vi "SSS_V3.0.vi"() -> ()   [LabVIEW 2017]
uses:
  <vilib>/DAQmx/write.llb/DAQmx Write (Analog 2D DBL NChan NSamp).vi
  <vilib>/DAQmx/read.llb/DAQmx Read (Analog 1D Wfm NChan NSamp).vi
  <vilib>/DAQmx/create/channels.llb/DAQmx Create Channel (AO-Voltage-Basic).vi
  <vilib>/DAQmx/create/channels.llb/DAQmx Create Channel (AI-Voltage-Basic).vi
  <vilib>/DAQmx/configure/timing.llb/DAQmx Timing (Sample Clock).vi
  <vilib>/DAQmx/miscellaneous.llb/DAQmx Fill In Error Info.vi
panel:
  out "배열":i32[](array[numeric])
  in  "physical channels":tag="Dev3/ao0:1" caption="송신 채널 설정"
  in  "Samplig Rate(RX)":dbl=1500000.0
  in  "RX time(sec)":dbl=0.1
  out "RX.CH2 2":waveform(dbl)(graph)
  out "RX.CH2":waveform(dbl)(graph)
  in  "Start Frequency(Hz)":dbl=430000.0 format="%#_6p"
  in  "Pulse length(sec)":dbl=4e-06 format="%#_6p"
  in  "sampling rate(TX)":dbl=3760000.0 caption="Sampling Rate(TX)" format="%#.2g"
  in  "STEP":i32=100
  in  "초기 위상":dbl format="%#_13g"
  in  "Bandwidth":dbl=40000.0 format="%#_6p"
  out "Hz/1STEP":dbl
  out "TX.CH1":waveform(dbl)(graph)
  out "TX Spectrum":cluster{"f0":dbl, "df":dbl, "magnitude":dbl[]}(graph)
  out "TX.CH 2":waveform(dbl)(graph)
  in  "수신 디바이스 이름":tag="Dev3"
  in  "수신 채널 설정":tag="Dev3/ai0:1"
  in  "Number of Sample":i32=150000 format="%#.0g"
  in  "송신 디바이스 이름":tag="Dev3"
  out "불리언 2":bool
  in  "Signal_Processing 2":bool
  out "CMD_PWD_DATA":i32=4
  in  "Signal_Processing":bool
  out "CMD_PWD":i32=7
  out "CMD_TVG":i32=6
  out "CMD_TVG_DATA":i32=4
  out "CMD_GAIN":i32=5
  out "CMD_GAIN_DATA":i32=255
  out "CMD_RANGE":i32=4
  out "CMD_RANGE_DATA":i32=100
  out "CMD_STOP":i32=3
  out "CMD_STOP_DATA":i32
  out "CMD_START":i32=2
  out "CMD_START_DATA":i32=1
  in  "port":u16=2500
  in  "address":string="30.0.1.18"
  in  "TCP/IP":bool
  in  "Server Closed":string="The server VI closed the connection."
  # "송신 신호 변조 설정"
  # "DAQ Max 설정"
  # "TCP/IP 소켓 통신 설정"
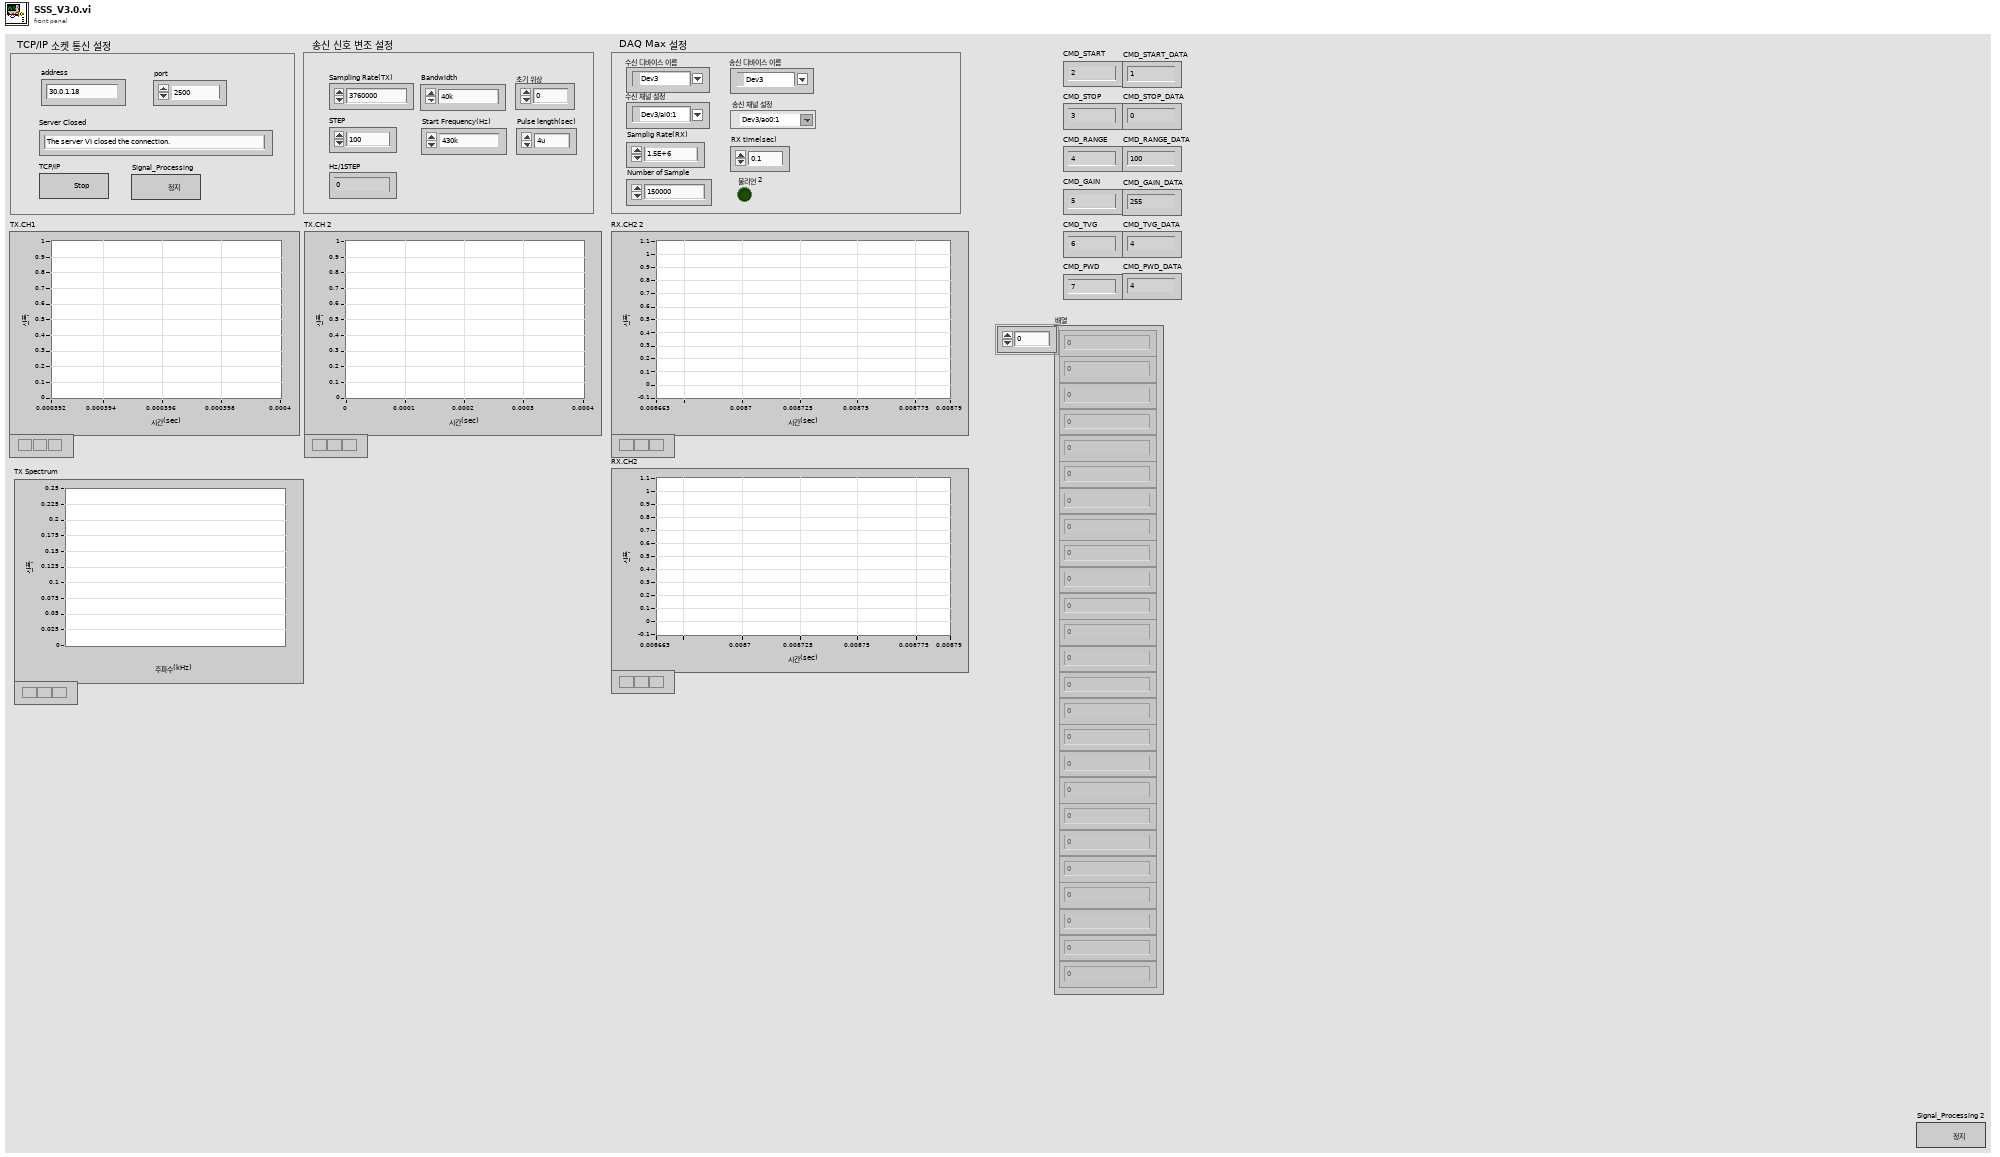
[diagram p1: front panel]
types:
  T1 = enum16{"Standard", "Buffered", "CRLF", "Immediate"}
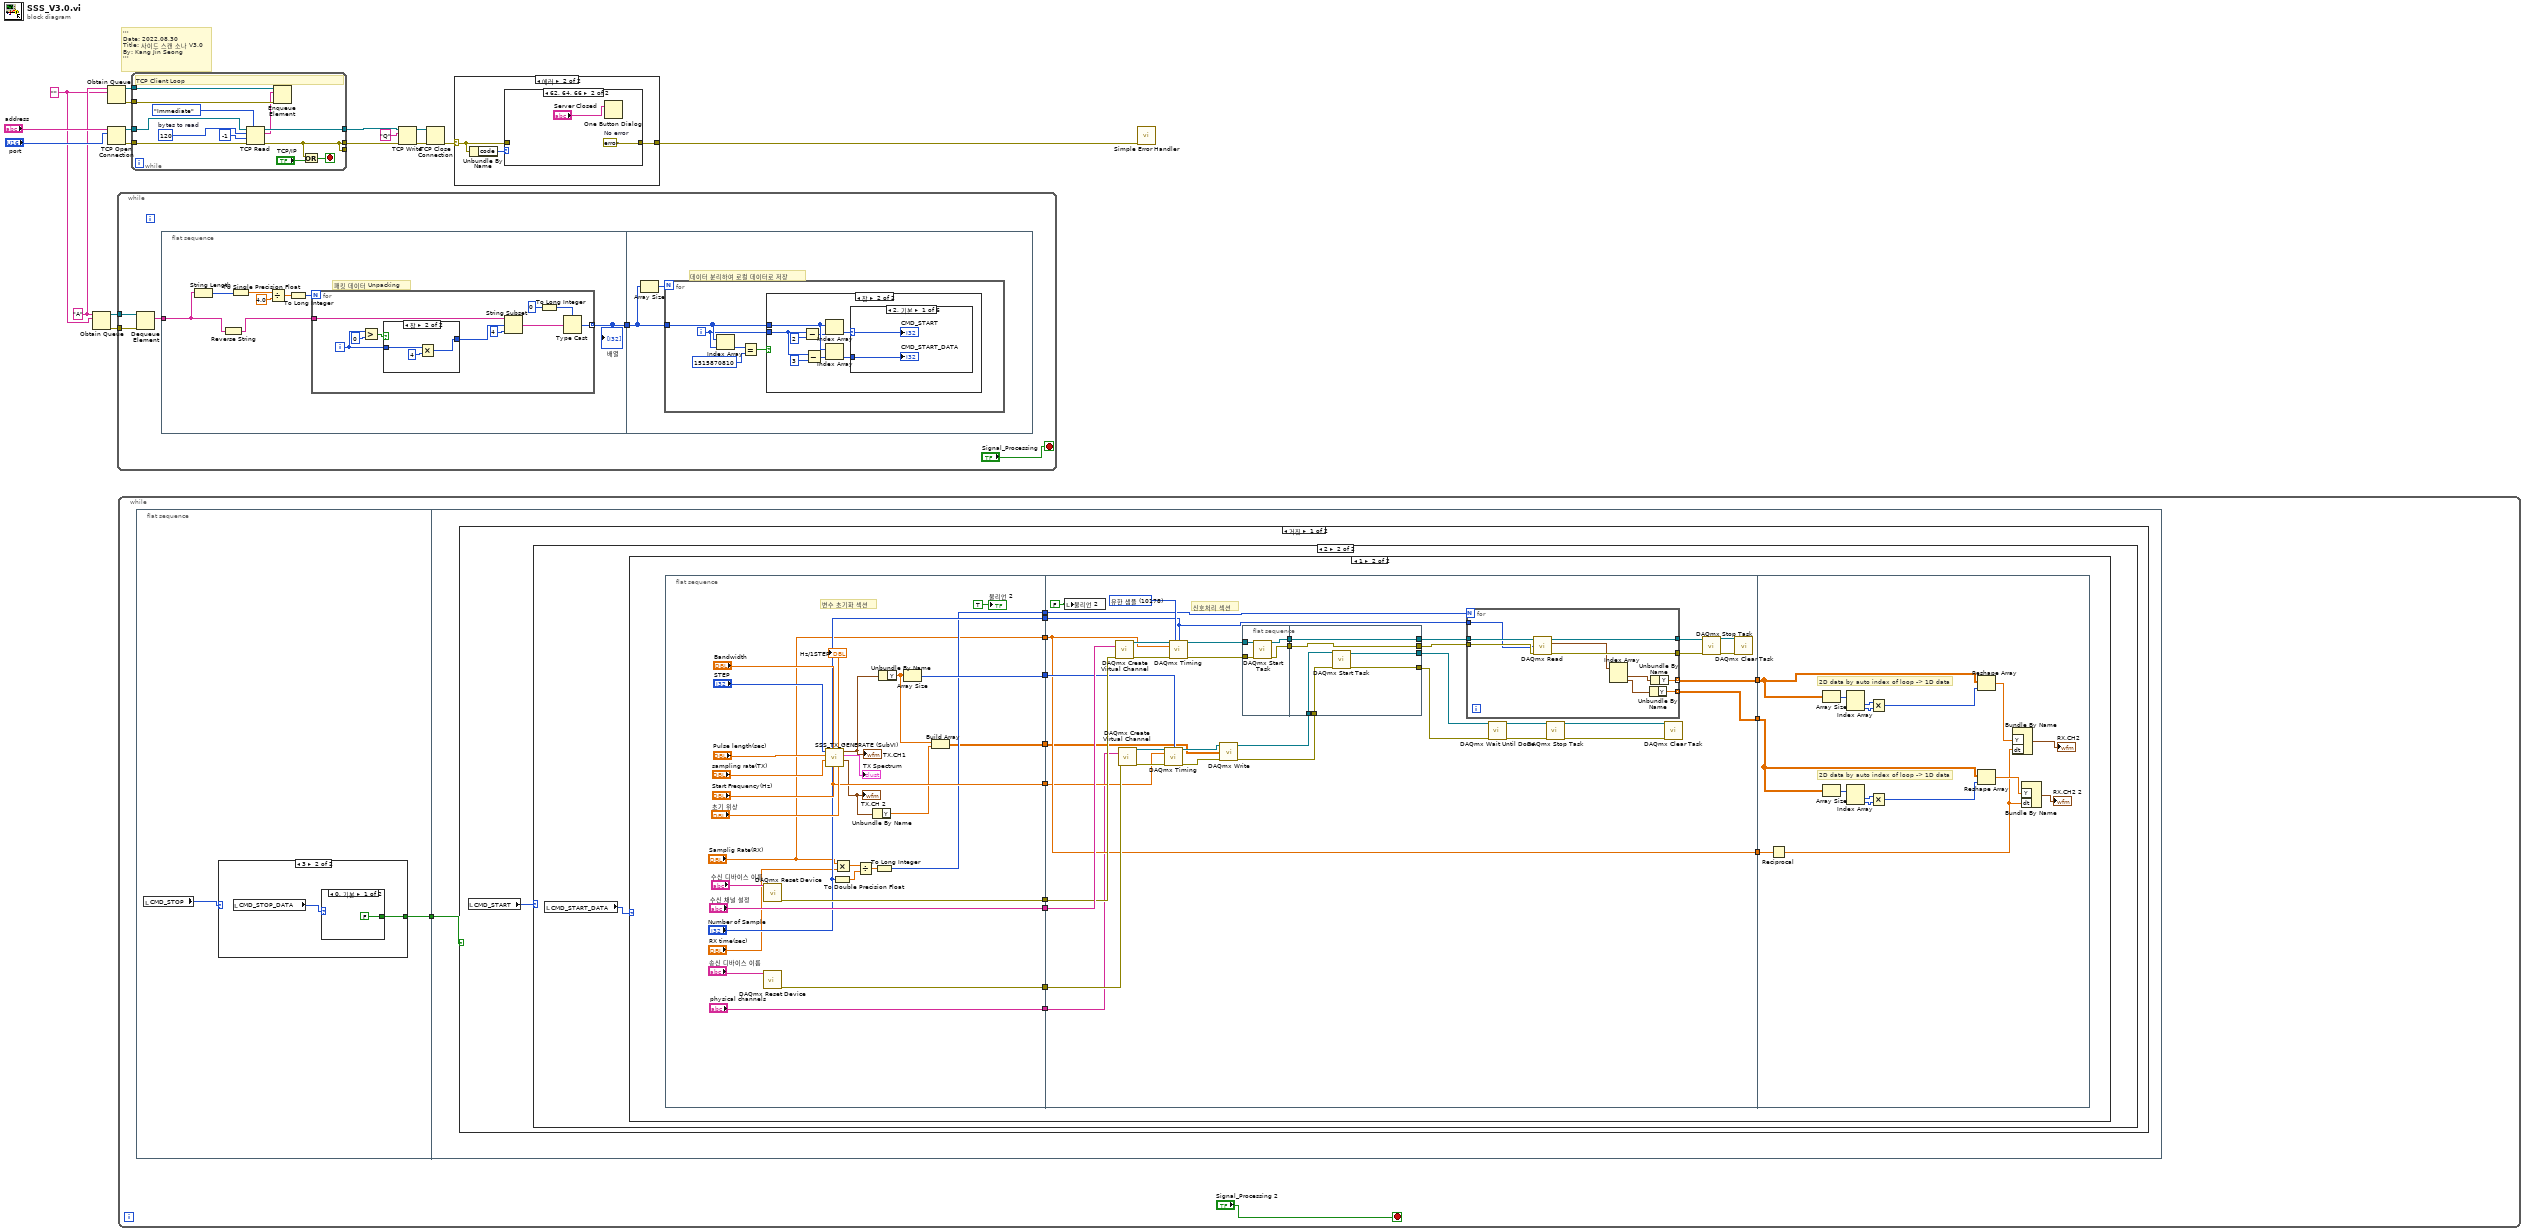
[diagram p0: block diagram]
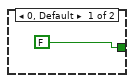
[diagram p2: hidden frame]
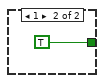
[diagram p3: hidden frame]
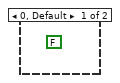
[diagram p4: hidden frame]
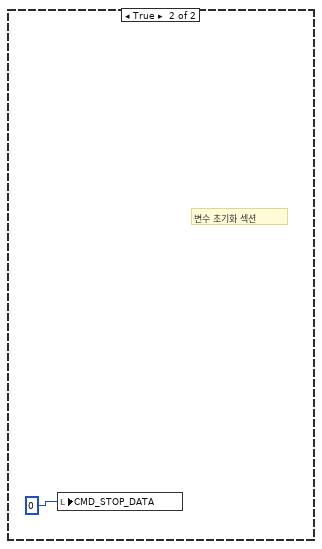
[diagram p6: hidden frame]
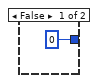
[diagram p7: hidden frame]
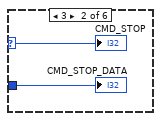
[diagram p9: hidden frame]
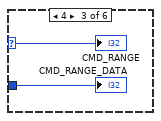
[diagram p10: hidden frame]
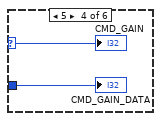
[diagram p11: hidden frame]
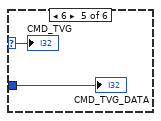
[diagram p12: hidden frame]
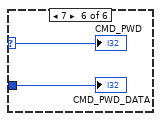
[diagram p13: hidden frame]
diagram:
  w1 = ""
  w4 = "A" ("이름(이름없음)")
  # "'''\nDate: 2022.08.30\nTitle: 사이드 스캔 소나 V3.0\nBy: Kang Jin Seong\n'''"
  n1 = Obtain Queue(name (unnamed)=w4, element data type=w1) -> (queue out=w3:refnum<queue>, error out=w2:errorcluster)  [unwired: 3 in, 1 out]
  n2 = Obtain Queue(name (unnamed)=w4, element data type=w1) -> (queue out=w6:refnum<queue>, error out=w5:errorcluster)  [unwired: 3 in, 1 out]
  n3 = TCP Open Connection(address="address", remote port or service name="port") -> (connection ID=w7:refnum<k5>, error out=w8:errorcluster)  [unwired: 3 in]
  n4 = while {
    tunnel: w3 -> [w21]
    tunnel: w2 -> [w20]
    stop <- "Signal_Processing" stop-if-true
    n5 = Dequeue Element(queue=w21, error in (no error)=w20) -> (element=w19:string)  [unwired: 1 in, 3 out]
    n6 = flat-sequence {
      tunnel: w19 -> [w24]
      tunnel: [w25] -> w22
      tunnel: w22 -> [w45]
      frame #0 {
        # "패킷 데이터 Unpacking"
        n7 = String Length(string=w24) -> (length=w30:i32)
        n8 = Reverse String(1:w24) -> (0:w23:string)
        n9 = To Single Precision Float(number=w30) -> (single precision float=w29:sgl)
        n10 = Divide(x=w29, y=sgl 4.0) -> (x/y=w27:sgl)
        n11 = To Long Integer(number=w27) -> (32bit integer=w26:i32)
        n12 = for {
          N: w26 -> [_]
          tunnel: w23 -> [w40]
          tunnel: [w37] -> w25 mode=indexing
          i -> [w32]
          n13 = Greater?(x=w32, y=0) -> (0:w34:bool)
          n14 = case shown="참" w34 {
            tunnel: [0 w42] -> w33
            tunnel: w32 -> [_ w44]
            frame False {
            }
            frame True {
              n15 = Multiply(x=w44, y=4) -> (x*y=w42:i32)
            }
          }
          n16 = String Subset(string=w40, offset (0)=w33, length (rest)=4 ("길이(나머지)")) -> (substring=w31:string)
          n17 = To Long Integer(number=0 ("숫자")) -> (32bit integer=w39:i32)
          n18 = Type Cast(type=w39, x=w31) -> (*(type *) &x=w37:i32)
        }
        "배열" <- w25
      }
      frame #1 {
        # "데이터 분리하여 로컬 데이터로 저장"
        n19 = Array Size(array=w45) -> (size(s)=w46:i32)
        n20 = for {
          N: w46 -> [_]
          tunnel: w45 -> [w48]
          i -> [w47]
          n21 = Index Array(array=w48, index=w47) -> (element=w51:i32)
          n22 = Equal?(x=w51, y=1515870810) -> (x = y?=w49:bool)
          n23 = case shown="참" w49 {
            tunnel: w48 -> [_ w58]
            tunnel: w47 -> [_ w54]
            frame False {
            }
            frame True {
              n24 = Subtract(x=w54, y=2) -> (x-y=w52:i32)
              n25 = Subtract(x=w54, y=3) -> (x-y=w55:i32)
              n26 = Index Array(array=w58, index=w52) -> (element=w59:i32)
              n27 = Index Array(array=w58, index=w55) -> (element=w57:i32)
              n28 = case shown="2, 기본" w59 {
                selector: w59 -> [w61 w63 w65 w67 w69 w71]
                tunnel: w57 -> [w60 w62 w64 w66 w68 w70]
                frame 2, Default {
                  "CMD_START" <- w61
                  "CMD_START_DATA" <- w60
                }
                frame 3 {
                  "CMD_STOP" <- w63
                  "CMD_STOP_DATA" <- w62
                }
                frame 4 {
                  "CMD_RANGE" <- w65
                  "CMD_RANGE_DATA" <- w64
                }
                frame 5 {
                  "CMD_GAIN" <- w67
                  "CMD_GAIN_DATA" <- w66
                }
                frame 6 {
                  "CMD_TVG" <- w69
                  "CMD_TVG_DATA" <- w68
                }
                frame 7 {
                  "CMD_PWD" <- w71
                  "CMD_PWD_DATA" <- w70
                }
              }
            }
          }
        }
      }
    }
  }
  n29 = while {
    stop <- "Signal_Processing 2" stop-if-true
    n30 = flat-sequence {
      tunnel: [w74] -> w72
      tunnel: w72 -> [w81]
      frame #0 {
        n31 = local read "CMD_STOP"() -> (w75:i32)
        n32 = case shown="3" w75 {
          tunnel: [FALSE w77] -> w74
          frame 0, Default {
          }
          frame 3 {
            n33 = local read "CMD_STOP_DATA"() -> (w78:i32)
            n34 = case shown="0, 기본" w78 {
              tunnel: [FALSE TRUE] -> w77
              frame 0, Default {
              }
              frame 1 {
              }
            }
          }
        }
      }
      frame #1 {
        n35 = case shown="거짓" w81 {
          frame False {
            n36 = local read "CMD_START"() -> (w82:i32)
            n37 = case shown="2" w82 {
              frame 0, Default {
                (unwired) FALSE
              }
              frame 2 {
                n38 = local read "CMD_START_DATA"() -> (w83:i32)
                n39 = case shown="1" w83 {
                  frame 0, Default {
                  }
                  frame 1 {
                    n40 = flat-sequence {
                      tunnel: ["Start Frequency(Hz)"] -> w96
                      tunnel: ["수신 채널 설정"] -> w95
                      tunnel: [w110] -> w94
                      tunnel: ["Samplig Rate(RX)"] -> w93
                      tunnel: ["Number of Sample"] -> w92
                      tunnel: [w108] -> w91
                      tunnel: [w106] -> w90
                      tunnel: [w105] -> w89
                      tunnel: [w100] -> w85
                      tunnel: ["physical channels"] -> w84
                      tunnel: [w138] -> w88
                      tunnel: w96 -> [w128]
                      tunnel: w95 -> [w136]
                      tunnel: w94 -> [w135]
                      tunnel: w93 -> [w130]
                      tunnel: w92 -> [w129]
                      tunnel: w91 -> [w133]
                      tunnel: w90 -> [w132]
                      tunnel: w89 -> [w131]
                      tunnel: [w130] -> w87
                      tunnel: [w127] -> w86
                      tunnel: w85 -> [w126]
                      tunnel: w84 -> [w125]
                      tunnel: w88 -> [w192]
                      tunnel: w87 -> [w191]
                      tunnel: w86 -> [w186]
                      frame #0 {
                        # "변수 초기화 섹션"
                        n41 = call <vilib>:"DAQmx Reset Device.vi"("device in"="송신 디바이스 이름") -> ("error out"=w105:errorcluster)  [unwired: 1 in, 13 out]
                        n42 = call <vilib>:"DAQmx Reset Device.vi"("device in"="수신 디바이스 이름") -> ("error out"=w110:errorcluster)  [unwired: 1 in, 13 out]
                        n43 = call "SSS_TX_GENERATE (SubVI).vi"("초기 위상"="초기 위상", "Start Frequency(Hz)"="Start Frequency(Hz)", "Bandwidth"="Bandwidth", "sampling rate"="sampling rate(TX)", "Pulse length(sec)"="Pulse length(sec)", "STEP"="STEP") -> ("TX.CH1 2"=w103:waveform(dbl), "TX Spectrum"=→"TX Spectrum":cluster{"f0":dbl, "df":dbl, "magnitude":dbl[]}, "TX.CH1"=w109:waveform(dbl), "Hz/1STEP"=→"Hz/1STEP":dbl)  [unwired: 2 in]
                        "TX.CH1" <- w109
                        "TX.CH 2" <- w103
                        n44 = To Double Precision Float(number="Number of Sample") -> (double precision float=w116:dbl)
                        n45 = Multiply(x="Samplig Rate(RX)", y="RX time(sec)") -> (x*y=w115:dbl)
                        n46 = Divide(x=w115, y=w116) -> (x/y=w117:dbl)
                        n47 = Unbundle By Name(w103) -> ("Y"=w101:dbl[])
                        n48 = To Long Integer(number=w117) -> (32bit integer=w106:i32)
                        n49 = Unbundle By Name(w109) -> ("Y"=w102:dbl[])
                        n50 = Array Size(array=w102) -> (size(s)=w108:i32)
                        n51 = Build Array(w102, w101) -> (w100:dbl[][])
                        "불리언 2" <- TRUE
                      }
                      frame #1 {
                        w134 = 10178 items=["유한 샘플"=10178, "연속 샘플"=10123, "하드웨어 타이밍에 의한 단일 포인트"=12522] ("sample mode")
                        # "신호처리 섹션"
                        n52 = local write "불리언 2"(FALSE) -> ()
                        n53 = call-poly <vilib>:"DAQmx Create Virtual Channel.vi"("physical channels"=w136, "error in"=w135) -> ("task out"=w159:refnum<k21>, "error out"=w160:errorcluster)  [unwired: 7 in, 5 out]
                        n54 = call-poly <vilib>:"DAQmx Create Virtual Channel.vi"("physical channels"=w125, "error in"=w131) -> ("task out"=w150:refnum<k21>, "error out"=w149:errorcluster)  [unwired: 7 in, 5 out]
                        n55 = call-poly <vilib>:"DAQmx Timing.vi"("task/channels in"=w150, "samples per channel"=w133, "rate"=w128, "error in"=w149) -> ("task out"=w147:refnum<k21>, "error out"=w148:errorcluster)  [unwired: 3 in, 7 out]
                        n56 = call-poly <vilib>:"DAQmx Timing.vi"("task/channels in"=w159, "sample mode"=w134, "samples per channel"=w129, "rate"=w130, "error in"=w160) -> ("task out"=w158:refnum<k21>, "error out"=w157:errorcluster)  [unwired: 2 in, 7 out]
                        n57 = call-poly <vilib>:"DAQmx Write.vi"("task/channels in"=w147, "data"=w126, "error in"=w148) -> ("task out"=w146:refnum<k21>, "error out"=w145:errorcluster)  [unwired: 10 in, 1 out]
                        n58 = flat-sequence {
                          tunnel: [w176] -> w162
                          tunnel: [w175] -> w161
                          tunnel: w158 -> [w174]
                          tunnel: w157 -> [w173]
                          tunnel: w162 -> [w182]
                          tunnel: [w182] -> w155
                          tunnel: [w181] -> w156
                          tunnel: w161 -> [w181]
                          tunnel: w146 -> [w180]
                          tunnel: w145 -> [w179]
                          tunnel: [w178] -> w140
                          tunnel: [w177] -> w139
                          frame #0 {
                            n59 = call <vilib>:"DAQmx Start Task.vi"("task/channels in"=w174, "error in"=w173) -> ("task out"=w175:refnum<k21>, "error out"=w176:errorcluster)  [unwired: 12 in]
                          }
                          frame #1 {
                            n60 = call <vilib>:"DAQmx Start Task.vi"("task/channels in"=w180, "error in"=w179) -> ("task out"=w178:refnum<k21>, "error out"=w177:errorcluster)  [unwired: 12 in]
                          }
                        }
                        n61 = for {
                          N: w132 -> [_]
                          tunnel: w156 -> [w172]
                          tunnel: w155 -> [w171]
                          tunnel: [w170] -> w154
                          tunnel: [w169] -> w151
                          tunnel: [w168] -> w138 mode=indexing
                          tunnel: w129 -> [w167]
                          tunnel: [w163] -> w127 mode=indexing
                          n62 = call-poly <vilib>:"DAQmx Read.vi"("task/channels in"=w172, "number of samples per channel"=w167, "error in"=w171) -> ("task out"=w169:refnum<k21>, "data"=w166:waveform(dbl)[], "error out"=w170:errorcluster)  [unwired: 10 out]
                          n63 = Index Array(array=w166) -> (element #1=w165:waveform(dbl), element #2=w164:waveform(dbl))  [unwired: 2 in]
                          n64 = Unbundle By Name(w164) -> ("Y"=w163:dbl[])
                          n65 = Unbundle By Name(w165) -> ("Y"=w168:dbl[])
                        }
                        n66 = call <vilib>:"DAQmx Wait Until Done.vi"("task/channels in"=w140, "error in"=w139) -> ("task out"=w142:refnum<k21>, "error out"=w141:errorcluster)  [unwired: 12 in]
                        n67 = call <vilib>:"DAQmx Stop Task.vi"("task/channels in"=w142, "error in"=w141) -> ("task out"=w144:refnum<k21>, "error out"=w143:errorcluster)  [unwired: 12 in]
                        n68 = call <vilib>:"DAQmx Clear Task.vi"("task in"=w144, "error in"=w143) -> ()  [unwired: 13 in, 1 out]
                        n69 = call <vilib>:"DAQmx Stop Task.vi"("task/channels in"=w151, "error in"=w154) -> ("task out"=w152:refnum<k21>, "error out"=w153:errorcluster)  [unwired: 12 out]
                        n70 = call <vilib>:"DAQmx Clear Task.vi"("task in"=w152, "error in"=w153) -> ()  [unwired: 14 out]
                      }
                      frame #2 {
                        # "2D data by auto index of loop -> 1D data"
                        # "2D data by auto index of loop -> 1D data"
                        n71 = Reciprocal(x=w191) -> (1/x=w184:dbl)
                        n72 = Array Size(array=w192) -> (size(s)=w196:i32[])
                        n73 = Array Size(array=w186) -> (size(s)=w188:i32[])
                        n74 = Index Array(array=w196) -> (element #1=w197:i32, element #2=w193:i32)  [unwired: 2 in]
                        n75 = Index Array(array=w188) -> (element #1=w189:i32, element #2=w187:i32)  [unwired: 2 in]
                        n76 = Multiply(x=w197, y=w193) -> (x*y=w198:i32)
                        n77 = Multiply(x=w189, y=w187) -> (x*y=w190:i32)
                        n78 = Reshape Array(w192, w198) -> (w195:dbl[])
                        n79 = Reshape Array(w186, w190) -> (w185:dbl[])
                        n80 = Bundle By Name("Y"=w195, "dt"=w184) -> (→"RX.CH2":waveform(dbl))  [unwired: 1 in]
                        n81 = Bundle By Name("Y"=w185, "dt"=w184) -> (→"RX.CH2 2":waveform(dbl))  [unwired: 1 in]
                      }
                    }
                  }
                }
              }
            }
          }
          frame True {
            # "변수 초기화 섹션"
            n82 = local write "CMD_STOP_DATA"(0) -> ()
          }
        }
      }
    }
  }
  n83 = while {
    tunnel: [w209] -> w16
    tunnel: [w202] -> w14
    tunnel: w8 -> [w207]
    tunnel: w7 -> [w206]
    tunnel: w6 -> [w205]
    tunnel: w5 -> [w204]
    tunnel: [w202] -> _
    stop <- w210 stop-if-true
    w211 = 120  # bytes to read
    # "TCP Client Loop"
    n84 = TCP Read(connection ID=w206, bytes to read=w211, error in (no error)=w207, 7:T1."Immediate" ("모드(standard)"), 9:-1 ("타임아웃 ms (25000)")) -> (connection ID out=w209:refnum<k5>, data out=w200:string, error out=w202:errorcluster)
    n85 = Enqueue Element(queue=w205, element=w200, error in (no error)=w204) -> ()  [unwired: 1 in, 3 out]
    n86 = Or(x=w202, y="TCP/IP") -> (x .or. y?=w210:bool)
  }
  n87 = TCP Write(connection ID=w16, data in="Q", error in (no error)=w14) -> (connection ID out=w17:refnum<k5>, error out=w15:errorcluster)  [unwired: 2 out]
  n88 = TCP Close Connection(connection ID=w17, error in (no error)=w15) -> (error out=w12:errorcluster)  [unwired: 1 in, 1 out]
  n89 = case shown="에러" w12 {
    selector: w12 -> [w212 w214]
    tunnel: [w212 w213] -> w11
    frame No Error {
    }
    frame Error {
      n90 = Unbundle By Name(w214) -> ("code"=w215:i32)
      n91 = case shown="62, 64, 66" w215 {
        tunnel: w214 -> [w216 _]
        tunnel: [w216 w218] -> w213
        frame Default {
        }
        frame 62, 64, 66 {
          w218 = errorcluster {"status"=FALSE, "code"=0, "source"=""}  # No error
          n92 = One Button Dialog(message="Server Closed") -> ()  [unwired: 1 in, 1 out]
        }
      }
    }
  }
  n93 = call <vilib>:"Simple Error Handler.vi"("error in (no error)"=w11) -> ()  [unwired: 4 in, 5 out]
